vi "MaxPIDIntegral.vi"(6 "Reset":bool, 7 "Output Range":cluster{"Max Output":dbl, "Min Output":dbl} {"Min Output" format="%.2f"; "Max Output" format="%.2f"}, 8 "dt (s)":dbl, 11 "Error":dbl) -> (3 "Integral":dbl)   [LabVIEW 2012]
panel:
  in  "Previous Error":dbl
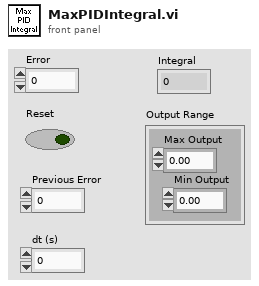
[diagram p1: front panel]
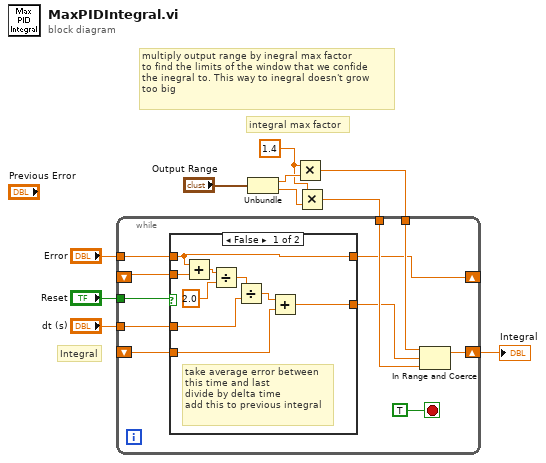
[diagram p0: block diagram]
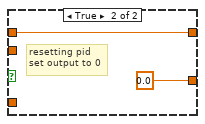
[diagram p2: hidden frame]
diagram:
  w3 = 1.4
  # "integral max factor"
  # "multiply output range by inegral max factor\nto find the limits of the window that we confide\nthe inegral to. This way to inegral doesn't grow \ntoo big"
  # "Integral"
  n1 = Unbundle("Output Range") -> ("Max Output"=w6:dbl, "Min Output"=w5:dbl)
  n2 = Multiply(x=w3, y=w6) -> (x*y=w2:dbl)
  n3 = Multiply(x=w3, y=w5) -> (x*y=w1:dbl)
  n4 = while {
    tunnel: "Error" -> [w20]
    tunnel: "Reset" -> [w19]
    tunnel: "dt (s)" -> [w18]
    shift-right: [w13] -> w7
    shift-left: _ -> [w17]
    tunnel: w2 -> [w16]
    tunnel: w1 -> [w15]
    shift-right: [w12] -> _
    shift-left: _ -> [w11]
    stop <- TRUE stop-if-true
    n5 = case shown="False" w19 {
      tunnel: w20 -> [w25 w31]
      tunnel: w18 -> [w30 _]
      tunnel: [w28 0.0] -> w14
      tunnel: w17 -> [w27 _]
      tunnel: [w25 w31] -> w12
      tunnel: w11 -> [w26 _]
      frame False {
        # "take average error between\nthis time and last\ndivide by delta time\nadd this to previous integral"
        n6 = Add(x=w25, y=w26) -> (x+y=w23:dbl)
        n7 = Divide(x=w23, y=2.0) -> (x/y=w24:dbl)
        n8 = Divide(x=w24, y=w30) -> (x/y=w29:dbl)
        n9 = Add(x=w29, y=w27) -> (x+y=w28:dbl)
      }
      frame True {
        # "resetting pid\nset output to 0"
      }
    }
    n10 = In Range and Coerce(upper limit=w16, x=w14, lower limit=w15) -> (coerced(x)=w13:dbl)  [unwired: 1 out]
  }
  "Integral" <- w7
